vi "XIPIN_MicroBlaze_9_5.vi"   [LabVIEW 2017]
doc: "The MicroBlaze 32 bit soft processor core, providing an instruction set optimized for embedded applications with many user-configurable options. MicroBlaze has many advanced architecture features like Instruction and Data-side cache with AXI interfaces, Floating-Point unit (FPU), Memory Management Unit (MMU), and fault tolerance support. It is highly recommended to create MicroBlaze systems within Vivado IP Integrator, to enable export to the Xilinx Software Development Kit (SDK) for software development.\n------------------------------------\n<b>Need License</b> : No\n<b>Interface</b> : AXI4 AXI4-Stream"
uses:
  <vilib>/rvi/XilinxIP/XIPIN_XNode/niFpgaXIPIN.xnode
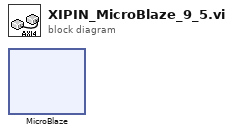
[diagram p0: block diagram]
diagram:
  n1 = xnode ("MicroBlaze")() -> ()
